vi "Create All Custom Chars.vi"(8 "error in (no error)":errorcluster, 9 "Custom Chars":T2, 11 "Char LCD in":refnum<class "Char LCD.lvclass">) -> (0 "error out":errorcluster, 3 "Char LCD out":refnum<class "Char LCD.lvclass">)   [LabVIEW 2020, in "CTI-Peripheral.lvlib" / "Char LCD.lvclass"]
uses:
  Char LCD.lvclass
  Custom Char.ctl
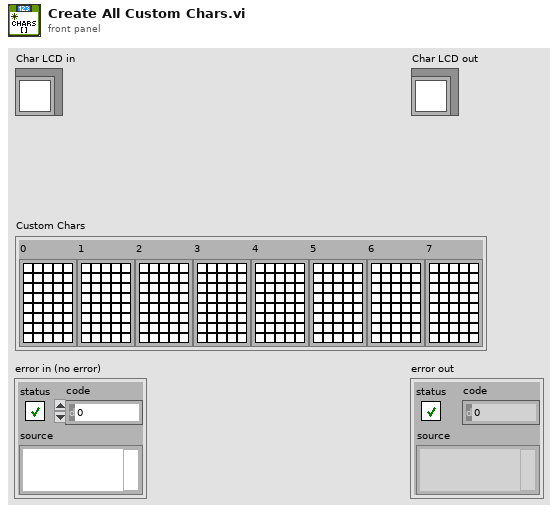
[diagram p1: front panel]
types:
  T1 = typedef "CTI-Peripheral.lvlib/Char LCD.lvclass/Custom Char.ctl" = bool[][]
  T2 = cluster{"0":T1, "1":T1, "2":T1, "3":T1, "4":T1, "5":T1, "6":T1, "7":T1}
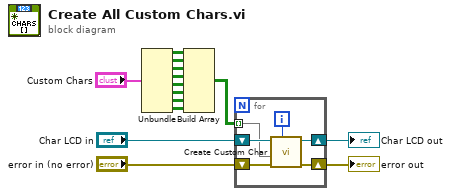
[diagram p0: block diagram]
diagram:
  n1 = Unbundle("Custom Chars") -> ("0"=w14:T1, "1"=w13:T1, "2"=w12:T1, "3"=w11:T1, "4"=w10:T1, "5"=w9:T1, "6"=w8:T1, "7"=w7:T1)
  n2 = Build Array(w14, w13, w12, w11, w10, w9, w8, w7) -> (w6:bool[][][])
  n3 = for {
    shift-right: [w19] -> w2
    shift-left: "error in (no error)" -> [w20]
    shift-right: [w17] -> w3
    shift-left: "Char LCD in" -> [w18]
    tunnel: w6 -> [w15] mode=indexing
    i -> [w16]
    n4 = call-dynamic "Create Custom Char.vi"("Char #"=w16, "error in (no error)"=w20, "Char"=w15, "Character LCD in"=w18) -> ("error out"=w19:errorcluster, "Character LCD out"=w17:refnum<class "Char LCD.lvclass">)  [unwired: 6 in]
  }
  "error out" <- w2
  "Char LCD out" <- w3
